vi "Exit.vi"(1 "board_sel":u32=6) -> ()   [LabVIEW 2015]
uses:
  ESLSCDLL.dll
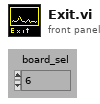
[diagram p1: front panel]
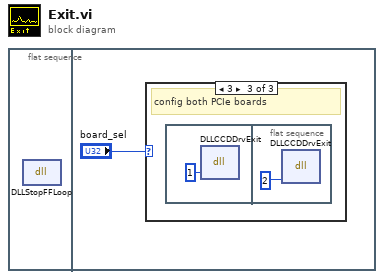
[diagram p0: block diagram]
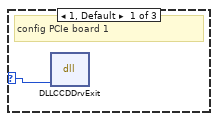
[diagram p2: hidden frame]
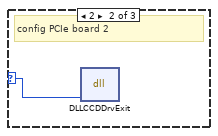
[diagram p3: hidden frame]
diagram:
  n1 = flat-sequence {
    frame #0 {
      n2 = dll-call lib="C:/Users/flori/Nextcloud/Dokumente/Stresing/Windows/lv64/board.vis/ESLSCDLL.dll" fn="DLLStopFFLoop"() -> ()  [unwired: 4 in, 2 out]
    }
    frame #1 {
      n3 = case shown="3" "board_sel" {
        selector: "board_sel" -> [w2 w3 _]
        frame 1, Default {
          # "config PCIe board 1"
          n4 = dll-call lib="C:/Users/flori/Nextcloud/Dokumente/Stresing/Windows/lv64/board.vis/ESLSCDLL.dll" fn="DLLCCDDrvExit"("drv"=w2) -> ()  [unwired: 5 in, 2 out]
        }
        frame 2 {
          # "config PCIe board 2"
          n5 = dll-call lib="C:/Users/flori/Nextcloud/Dokumente/Stresing/Windows/lv64/board.vis/ESLSCDLL.dll" fn="DLLCCDDrvExit"("drv"=w3) -> ()  [unwired: 5 in, 2 out]
        }
        frame 3 {
          # "config both PCIe boards"
          n6 = flat-sequence {
            frame #0 {
              n7 = dll-call lib="C:/Users/flori/Nextcloud/Dokumente/Stresing/Windows/lv64/board.vis/ESLSCDLL.dll" fn="DLLCCDDrvExit"("drv"=u32 1) -> ()  [unwired: 5 in, 2 out]
            }
            frame #1 {
              n8 = dll-call lib="C:/Users/flori/Nextcloud/Dokumente/Stresing/Windows/lv64/board.vis/ESLSCDLL.dll" fn="DLLCCDDrvExit"("drv"=u32 2) -> ()  [unwired: 5 in, 2 out]
            }
          }
        }
      }
    }
  }
